vi "CNT Length.vi"(10 "m-nm l":dbl, 11 "Length of CNTs":dbl) -> (3 "Numeric":dbl)   [LabVIEW 2020]
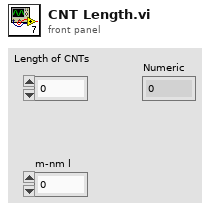
[diagram p1: front panel]
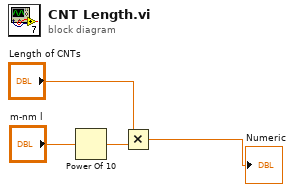
[diagram p0: block diagram]
diagram:
  n1 = Power Of 10(x="m-nm l") -> (10^x=w2:dbl)
  n2 = Multiply(x="Length of CNTs", y=w2) -> (x*y=→"Numeric":dbl)
